vi "Get Axis Motion Status_CK.vi"(4 "error in (no error)":errorcluster, 6 "Axis (1)":i32=1 min=1 max=3, 7 "VISA resource name":refnum<visa-resource-name>) -> (0 "error out":errorcluster, 2 "Motion Done":bool, 3 "VISA resource name out":refnum<visa-resource-name>)   [LabVIEW 2013]
doc: "Reads the motion status for the specified axis. This command can be used to monitor Homing, absolute and relative displacement move completion status."
uses:
  <vilib>/Utility/error.llb/whitespace.ctl
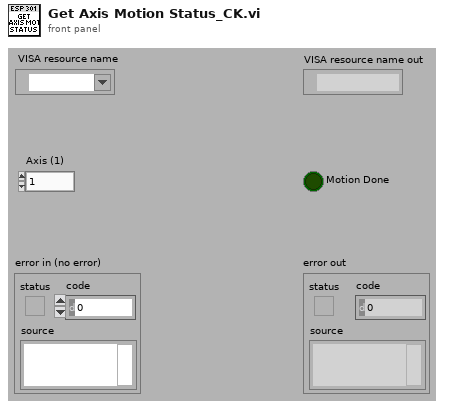
[diagram p1: front panel]
types:
  T1 = typedef "whitespace.ctl" = u16
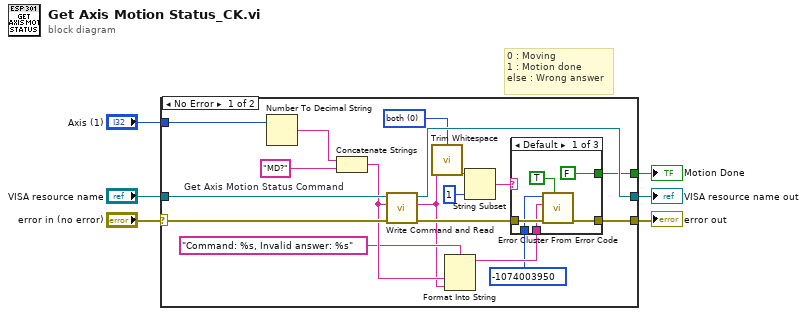
[diagram p0: block diagram]
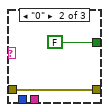
[diagram p2: hidden frame]
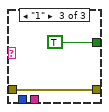
[diagram p3: hidden frame]
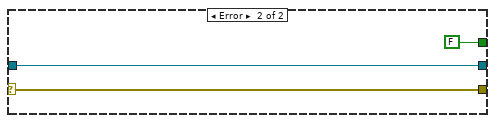
[diagram p4: hidden frame]
diagram:
  # "0 : Moving\n1 : Motion done\nelse : Wrong answer"
  n1 = case shown="No Error" "error in (no error)" {
    selector: "error in (no error)" -> [w23 w37]
    tunnel: [w16 w37] -> w5
    tunnel: "VISA resource name" -> [w24 w36]
    tunnel: [w15 w36] -> w3
    tunnel: "Axis (1)" -> [w21 _]
    tunnel: [w14 FALSE ("Motion Done")] -> w1
    frame No Error {
      w7 = T1 0 items=["both", "start of string", "end of string"] ("location (both)")
      w20 = "MD?"  # Get Axis Motion Status Command
      n2 = Number To Decimal String(number=w21) -> (decimal integer string=w22:string)  [unwired: 1 in]
      n3 = Concatenate Strings(w22, w20) -> (w13:string)
      n4 = call <instrlib>:"Write Command and Read.vi"("error in (no error)"=w23, "Command"=w13, "VISA resource name"=w24) -> ("error out"=w17:errorcluster, "Returned string"=w9:string, "VISA resource name out"=w15:refnum<visa-resource-name>)  [unwired: 4 in]
      n5 = call <vilib>:"Trim Whitespace.vi"("string"=w9, "location (both)"=w7) -> ("trimmed string"=w8:string)
      n6 = Format Into String(format string="Command: %s, Invalid answer: %s" ("error message (\"\")"), w13, w9) -> (resulting string=w11:string)  [unwired: 2 in, 1 out]
      n7 = String Subset(string=w8, length (rest)=1 ("longueur (reste)")) -> (substring=w18:string)  [unwired: 1 in]
      n8 = case shown="Default" w18 {
        tunnel: w17 -> [w27 w32 w34]
        tunnel: [w29 w32 w34] -> w16
        tunnel: [FALSE ("Motion Done") FALSE ("Motion Done") TRUE ("Motion Done")] -> w14
        tunnel: w11 -> [w26 _ _]
        tunnel: -1074003950 ("error code (0)") -> [w25 _ _]
        frame Default {
          n9 = call <vilib>:"Error Cluster From Error Code.vi"("show call chain? (False)"=TRUE, "error in (no error)"=w27, "error message (\"\")"=w26, "error code (0)"=w25) -> ("error out"=w29:errorcluster)  [unwired: 5 in]
        }
        frame "0" {
        }
        frame "1" {
        }
      }
    }
    frame Error {
    }
  }
  "error out" <- w5
  "VISA resource name out" <- w3
  "Motion Done" <- w1
